vi "ActionVIOnCompile.vi"(8 "error in (no error)":errorcluster, 11 "Device Item Ref in":T1 format="%.0x") -> (0 "error out":errorcluster)   [LabVIEW 2019, in "Diagnostics Addon System Explorer.lvlib"]
uses:
  Diagnostics Addon System Explorer.lvlib
  <vilib>/NI VeriStand/Custom Device API/Custom Device Item Ref.ctl
  Addon Shared/SubVIs/Constants.vi
  <vilib>/NI VeriStand/Custom Device API/Set Item Property (Variant).vi
  <vilib>/NI VeriStand/Custom Device API/Custom Device API.lvlib
  Addon Shared/Diagnostics Addon Shared.lvlib
  <vilib>/NI/NIVS Inline Async API/_Data Access System Explorer/Data Access System Explorer.lvlib
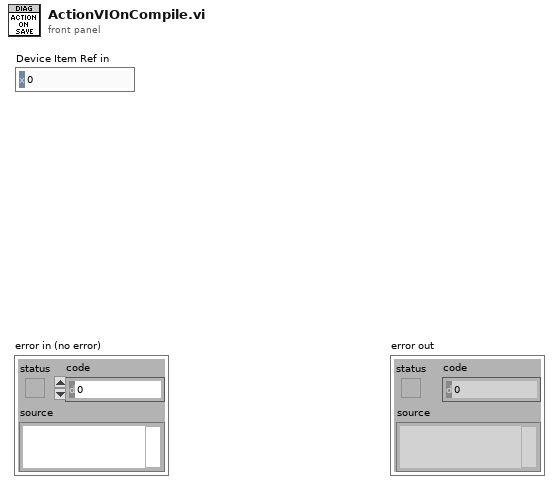
[diagram p1: front panel]
types:
  T1 = typedef "Custom Device API.lvlib/Custom Device Item Ref.ctl" = u64
  T2 = cluster{"Name":string, "Type":enum16{"Output/Write", "Input/Read", "Input/ReadWrite"}, "VS Refs":T1[]}[]
  T3 = typedef "Diagnostics Addon Shared.lvlib/SysDef.Compile.ctl" = cluster{"Name":string, "CAN":T4, "986x":T8, "Reads":T9[], "Frames Lookup":variant, "Writes":T9[], "DPIDs":T12[], "DPID Lookup":variant, "DTC":T14, "Created DTCs":u32, "Polls":T16[], "Service Channels Status Lookup":variant, "Trigger Lookup":variant, "Security":T17}
  T4 = typedef "Diagnostics Addon Shared.lvlib/CAN.ctl" = cluster{"Interface":T5, "Baud Rate":u64, "Diagnostic Protocol":T6, "Transport Protocol":T7, "Transmit ID":u32, "Receive ID":u32, "Transmit Extension":u8, "Receive Extension":u8, "Receive UUDT ID":u32, "Enable Stream":bool, "VW TP Channel ID":u32, "Fill Frame":bool, "Fill Byte":u8, "Termination":bool, "LIN Cluster":refnum<k21>, "NAD":u8, "IO Mode":u32, "Max DLC":u16, "FD Baud Rate":u64, "Timeout":u32}
  T5 = typedef "Diagnostics Addon Shared.lvlib/CAN.Interface.ctl" = string
  T6 = typedef "Diagnostics Addon Shared.lvlib/Protocol.ctl" = enum16{"GMLAN", "KWP-2000", "UDS", "User-Defined"}
  T7 = typedef "Diagnostics Addon Shared.lvlib/Transport.ctl" = enum16{"ISO TP - Normal Mode", "ISO TP - Mixed Mode", "VW TP 2.0", "Diagnostics on IP", "ISO TP LIN"}
  T8 = typedef "Diagnostics Addon Shared.lvlib/986x.ctl" = cluster{"Enable":bool, "RIO Device":string, "Bitfile":path}
  T9 = typedef "Diagnostics Addon Shared.lvlib/Frame.Compile.ctl" = cluster{"ID":u32, "Type":T10, "Signals":T11[]}
  T10 = typedef "Diagnostics Addon Shared.lvlib/Type.ctl" = enum16{"DID", "CDID", "PID", "CPID", "Read Memory", "Write Memory", "IO Control", "Routine Start", "Routine Request", "Routine Stop", "User Defined", "DTC Control", "Clear DTCs", "Read DTCs", "Start DTCs", "DTC Change Count", "Tester Present", "Unlock ECU", "Reset ECU", "Diag Session Control", "Communication Control", "DPID Control", "Poll Control", "Diag CAN Control"}
  T11 = typedef "Diagnostics Addon Shared.lvlib/Signal.ctl" = cluster{"Start Bit":u32, "Length":u32, "Scaling Factor":dbl, "Scaling Offset":dbl, "Minimum":dbl, "Maximum":dbl, "Data Type":u32, "Byte Order":u32, "Default Value":dbl, "Name":string, "Units":string}
  T12 = typedef "Diagnostics Addon Shared.lvlib/DPID.ctl" = cluster{"DPID ID":u8, "Speed":T13, "PIDs":u16[]}
  T13 = typedef "Diagnostics Addon Shared.lvlib/DPID.Rate.ctl" = enum16{"Slow", "Medium", "Fast"}
  T14 = typedef "Diagnostics Addon Shared.lvlib/DTC.Settings.ctl" = cluster{"Descriptor":T15, "Value.Code":dbl[], "Value.String":string[], "Value.J2012String":string[], "Status.Code":dbl[], "Status.String":string[]}
  T15 = typedef "Diagnostics Addon Shared.lvlib/DTC.Descriptor.ctl" = cluster{"DTC Byte Length":i32, "Status Byte Length":i32, "Add Data Byte Length":i32, "Byte Order":enum16{"Motorola", "Intel"}}
  T16 = typedef "Diagnostics Addon Shared.lvlib/Poll.Compiled.ctl" = cluster{"Speed":T13, "DID IDs":u32[], "PID IDs":u32[]}
  T17 = typedef "Diagnostics Addon Shared.lvlib/Security.ctl" = cluster{"Type":T18, "Source DLL Path":path, "Target DLL Path":path, "Security Level":u8}
  T18 = typedef "Diagnostics Addon Shared.lvlib/Security.Type.ctl" = enum16{"None", "DLL", "MasterKey"}
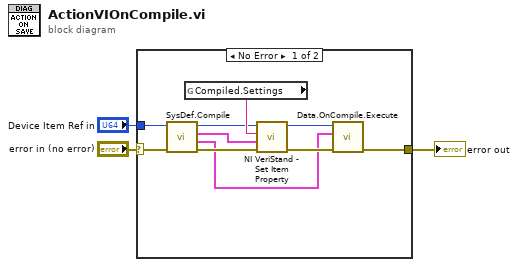
[diagram p0: block diagram]
diagram:
  n1 = case shown="No Error" "error in (no error)" {
    selector: "error in (no error)" -> [w4 w14]
    tunnel: [w7 w14] -> w2
    tunnel: "Device Item Ref in" -> [w13 _]
    frame No Error {
      n2 = call "SysDef.Compile.vi"("error in (no error)"=w4, "Device Reference in"=w13) -> ("error out"=w9:errorcluster, "Refs"=w5:T2, "VS References"=w12:T3, "Device Reference out"=w10:T1)  [unwired: 6 in]
      n3 = global read "Constants.vi" "Compiled.Settings"() -> (w11:string)
      n4 = call-poly <vilib>:"NI VeriStand - Set Item Property.vi"("error in (no error)"=w9, "Value"=w12, "Property Name"=w11, "Item Ref in"=w10) -> ("error out"=w8:errorcluster, "Item Ref out"=w6:T1)  [unwired: 5 in, 1 out]
      n5 = call <vilib>:"Data.OnCompile.Execute.vi"("error in"=w8, "VS Ref Groups"=w5, "Custom Device Ref"=w6) -> ("error out"=w7:errorcluster)  [unwired: 7 in, 1 out]
    }
    frame Error {
    }
  }
  "error out" <- w2
